vi "Riffle Array (I32).vi"(10 "seed":i32=-1, 11 "X":i32[](array[numeric])) -> (0 "error":i32, 2 "Riffled Index":i32[](array[numeric]), 3 "Riffled {X}":i32[](array[numeric]))   [LabVIEW 2014, in "NI_AALBase.lvlib"]
doc: "Riffles the elements in the input array <B>X</B>. Wire data to the <B>X</B> input to determine the polymorphic instance to use or manually select the instance."
uses:
  NI_AALBase.lvlib
  lvanlys.dll
panel:
  # "Riffle Array (I32)"
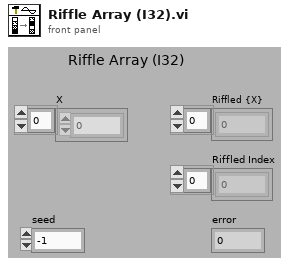
[diagram p1: front panel]
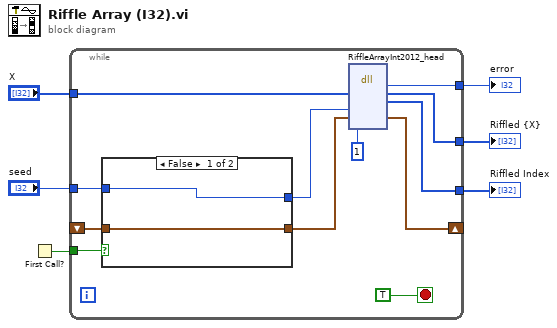
[diagram p0: block diagram]
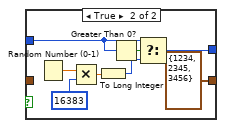
[diagram p2: hidden frame]
diagram:
  n1 = First Call?() -> (First Call?: T/F=w6:bool)
  n2 = while {
    tunnel: "seed" -> [w17]
    shift-right: [w9] -> _
    shift-left: _ -> [w15]
    tunnel: w6 -> [w16]
    tunnel: [w14] -> w3
    tunnel: [w13] -> w5
    tunnel: "X" -> [w12]
    tunnel: [w8] -> w1
    stop <- TRUE stop-if-true
    n3 = case shown="False" w16 {
      tunnel: w15 -> [w20 _]
      tunnel: [w20 cluster{"xSeed":i32, "ySeed":i32, "zSeed":i32} {"xSeed"=1234, "ySeed"=2345, "zSeed"=3456} ("RNGState")] -> w11
      tunnel: [w19 w26] -> w10
      tunnel: w17 -> [w19 w27]
      frame False {
      }
      frame True {
        n4 = Random Number (0-1)() -> (number: 0 to 1=w24:dbl)
        n5 = Multiply(x=w24, y=16383 ("x")) -> (x*y=w25:dbl)
        n6 = To Long Integer(number=w25) -> (32bit integer=w23:i32)
        n7 = Greater Than 0?(x=w27) -> (x > 0?=w28:bool)
        n8 = Select(t=w27, s=w28, f=w23) -> (s? t:f=w26:i32)
      }
    }
    n9 = dll-call lib="C:/Program Files (x86)/National Instruments/LabVIEW 2014/resource/lvanlys.*" fn="RiffleArrayInt2012_head"("riffle"=w12, "seed"=w10, "rngState"=w11, "option"=1) -> ("return type"=w14:i32, "riffle"=w13:i32[], "riffleIndx"=w8:i32[], "rngState"=w9:cluster{"xSeed":i32, "ySeed":i32, "zSeed":i32})  [unwired: 6 in, 2 out]
  }
  "Riffled {X}" <- w5
  "error" <- w3
  "Riffled Index" <- w1
